vi "CreateCommunication.vi"(8 "error in (no error)":errorcluster) -> (0 "error out":errorcluster, 3 "Message Queues out":T1)   [LabVIEW 2017, in "Server.lvlib" / "Message Queue.lvlib"]
doc: "Creates all Queues and User Events and stores them in References Cluster."
uses:
  Message Queue.lvlib
  CommReferences.ctl
  MessageCluster.ctl
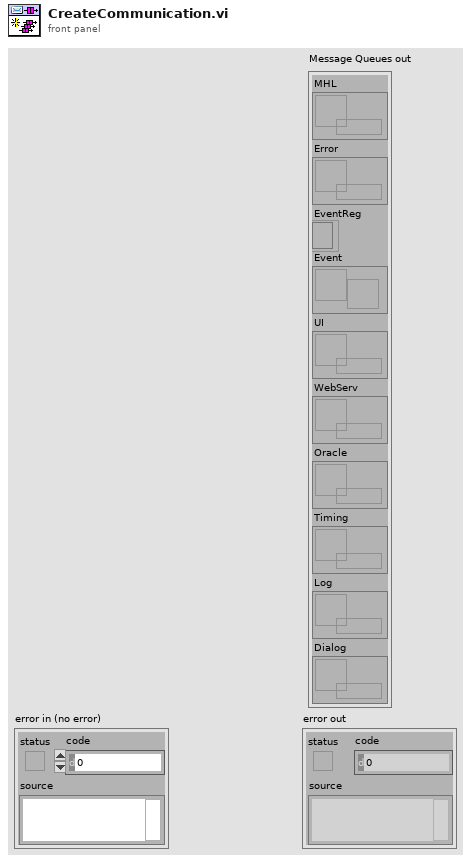
[diagram p1: front panel]
types:
  T1 = typedef "Server.lvlib/Message Queue.lvlib/CommReferences.ctl" = cluster{"MHL":refnum<queue>, "Error":refnum<queue>, "EventReg":refnum<event-registration>, "Event":refnum<user-event>, "UI":refnum<queue>, "WebServ":refnum<queue>, "Oracle":refnum<queue>, "Timing":refnum<queue>, "Log":refnum<queue>, "Dialog":refnum<queue>}
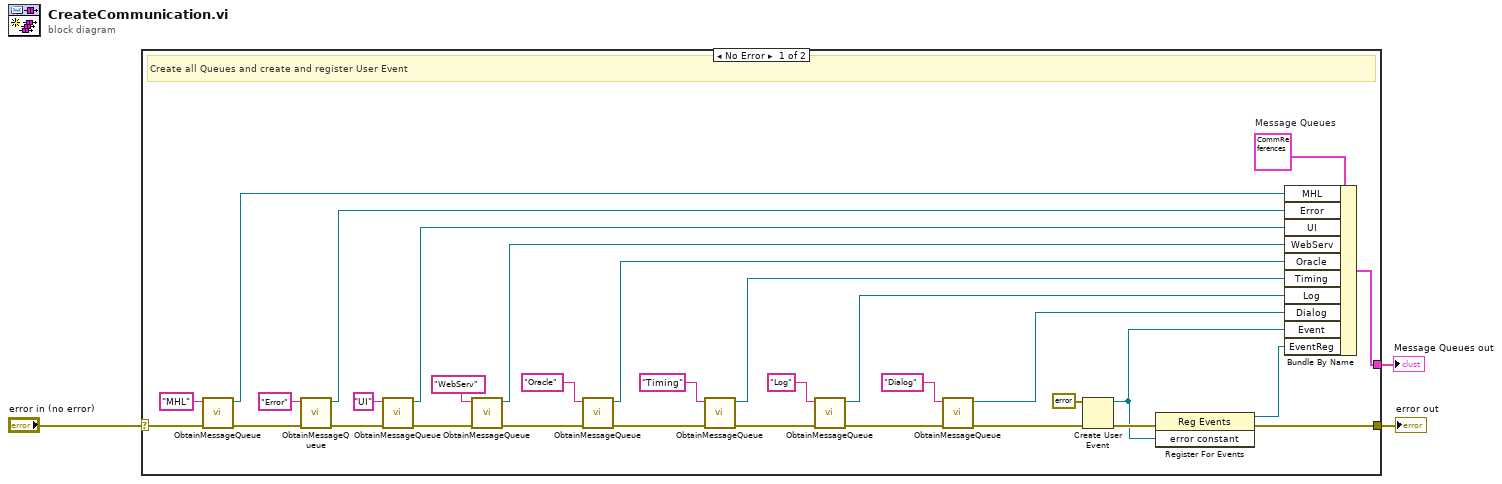
[diagram p0: block diagram]
diagram:
  n1 = case shown="No Error" "error in (no error)" {
    selector: "error in (no error)" -> [w33 w36]
    tunnel: [w24 w36] -> w3
    tunnel: [w34 _] -> w2
    frame No Error {
      w35 = T1 {"MHL"=refnum, "Error"=refnum, "EventReg"=refnum, "Event"=refnum, "UI"=refnum, "WebServ"=refnum, "Oracle"=refnum, "Timing"=refnum, "Log"=refnum, "Dialog"=refnum}  # Message Queues
      # "Create all Queues and create and register User Event"
      n2 = call "ObtainMessageQueue.vi"("error in (no error)"=w33, "Name"="MHL") -> ("error out"=w32:errorcluster, "Message Queue"=w31:refnum<queue>)  [unwired: 8 in]
      n3 = call "ObtainMessageQueue.vi"("error in (no error)"=w32, "Name"="Error") -> ("error out"=w27:errorcluster, "Message Queue"=w28:refnum<queue>)  [unwired: 8 in]
      n4 = call "ObtainMessageQueue.vi"("error in (no error)"=w27, "Name"="UI") -> ("error out"=w23:errorcluster, "Message Queue"=w22:refnum<queue>)  [unwired: 8 in]
      n5 = call "ObtainMessageQueue.vi"("error in (no error)"=w23, "Name"="WebServ") -> ("error out"=w18:errorcluster, "Message Queue"=w19:refnum<queue>)  [unwired: 8 in]
      n6 = call "ObtainMessageQueue.vi"("error in (no error)"=w18, "Name"="Oracle") -> ("error out"=w14:errorcluster, "Message Queue"=w17:refnum<queue>)  [unwired: 8 in]
      n7 = call "ObtainMessageQueue.vi"("error in (no error)"=w14, "Name"="Timing") -> ("error out"=w11:errorcluster, "Message Queue"=w13:refnum<queue>)  [unwired: 8 in]
      n8 = call "ObtainMessageQueue.vi"("error in (no error)"=w11, "Name"="Log") -> ("error out"=w8:errorcluster, "Message Queue"=w10:refnum<queue>)  [unwired: 8 in]
      n9 = call "ObtainMessageQueue.vi"("error in (no error)"=w8, "Name"="Dialog") -> ("error out"=w7:errorcluster, "Message Queue"=w4:refnum<queue>)  [unwired: 8 in]
      n10 = Create User Event(user event datatype=errorcluster {"status"=FALSE, "code"=0, "source"=""} ("error constant"), error in=w7) -> (user event=w5:refnum<user-event>, error out=w26:errorcluster)
      n11 = register-events(error in=w26, w5) -> (reference out=w6:refnum<event-registration>, error out=w24:errorcluster)  [unwired: 1 in]
      n12 = Bundle By Name(cluster=w35, "MHL"=w31, "Error"=w28, "UI"=w22, "WebServ"=w19, "Oracle"=w17, "Timing"=w13, "Log"=w10, "Dialog"=w4, "Event"=w5, "EventReg"=w6) -> (w34:T1)
    }
    frame Error {
    }
  }
  "Message Queues out" <- w2
  "error out" <- w3
